vi "FGV_OBJ_login.vi"(6 "login_refnums":T1, 7 "options":T2, 8 "error_in":errorcluster, 9 "access_level_in":i32, 10 "username_in":string, 11 "ID_in":string) -> (0 "error_out":errorcluster, 1 "access_level_out":i32, 2 "username_out":string, 3 "ID_out":string, 5 "Login read active?":bool)   [LabVIEW 2020]
uses:
  FGV_OBJ_login.ctl
  OBJ_login_refnums.ctl
  test_button/FGV_OBJ_test_button.ctl
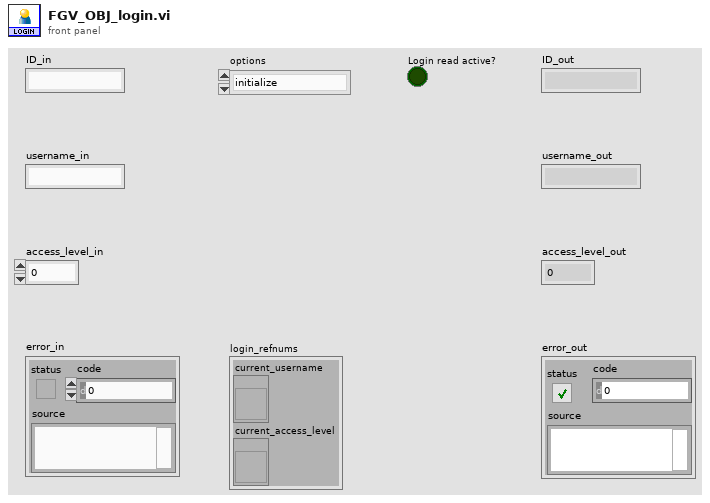
[diagram p1: front panel]
types:
  T1 = typedef "OBJ_login_refnums.ctl" = cluster{"current_username":refnum<vi>, "current_access_level":refnum<vi>}
  T2 = typedef "FGV_OBJ_login.ctl" = enum16{"initialize", "start_login_read", "end_login_read", "login", "logout", "get_login_info"}
  T3 = typedef "FGV_OBJ_test_button.ctl" = enum16{"initialize", "set_new_login", "set_message", "enable", "disable", "disable_gray", "translate", "set_scan_tooling", "get_scan_tooling"}
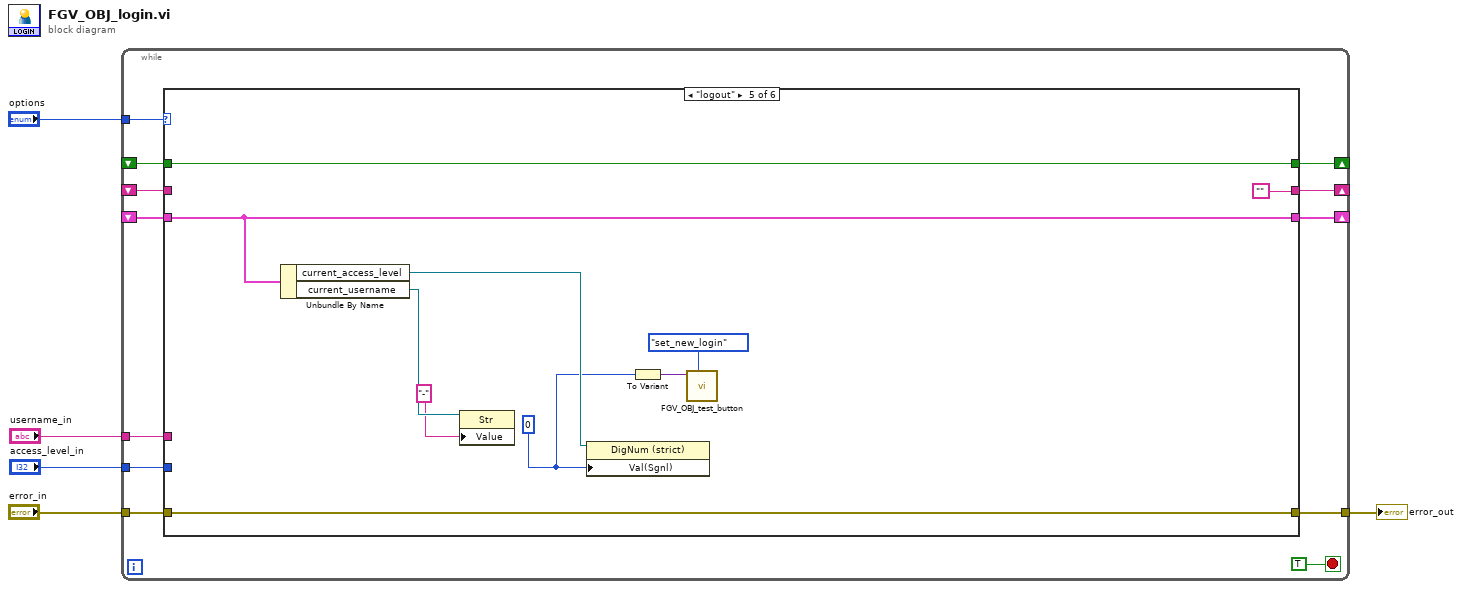
[diagram p0: block diagram]
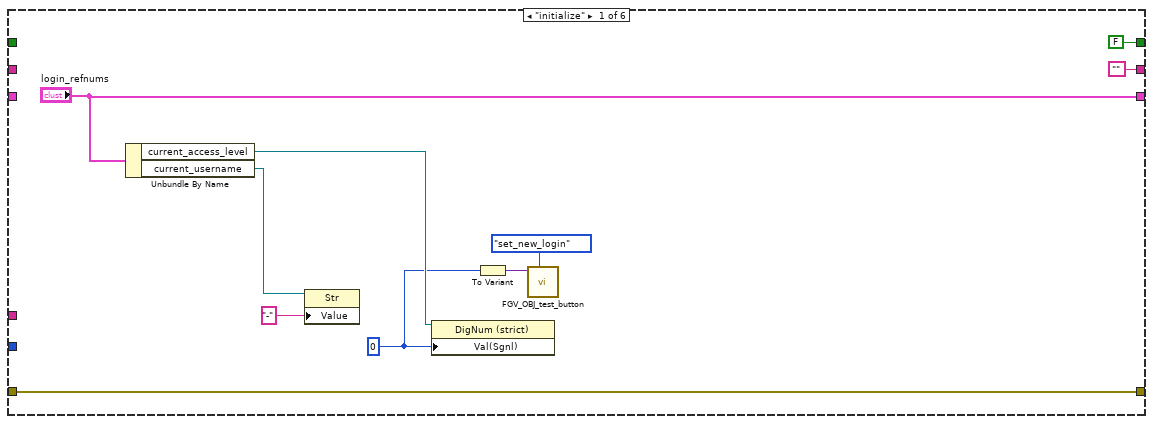
[diagram p2: hidden frame]
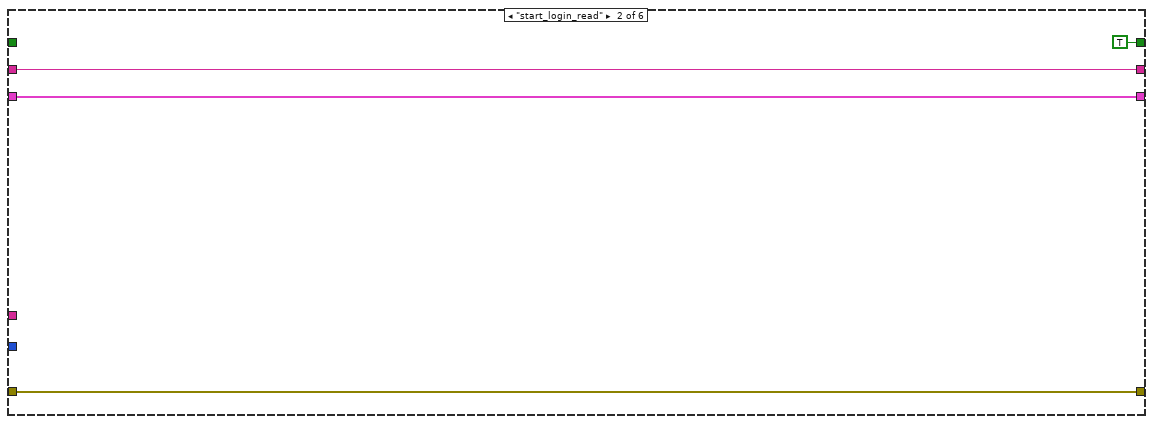
[diagram p3: hidden frame]
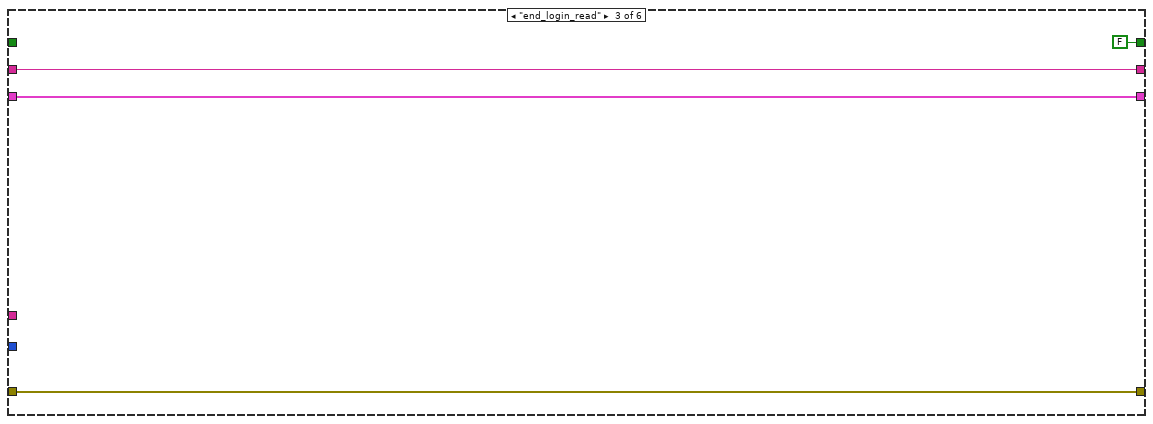
[diagram p4: hidden frame]
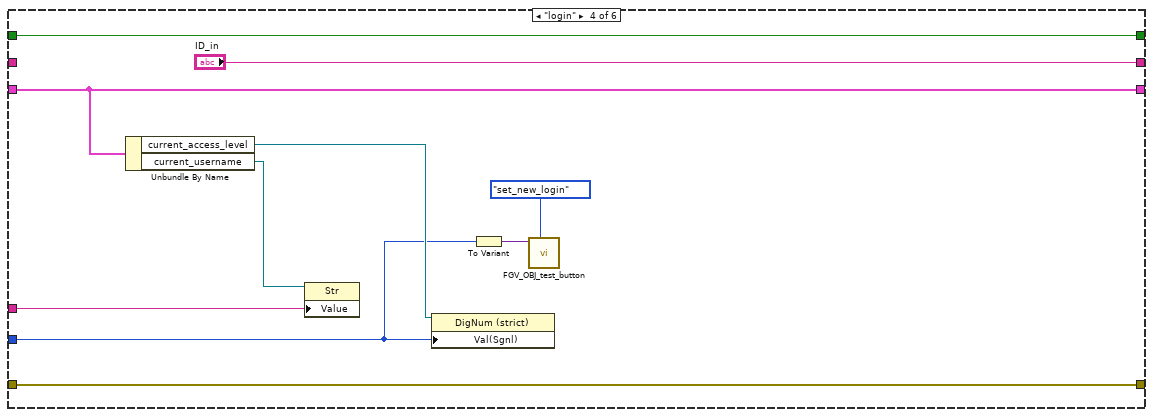
[diagram p5: hidden frame]
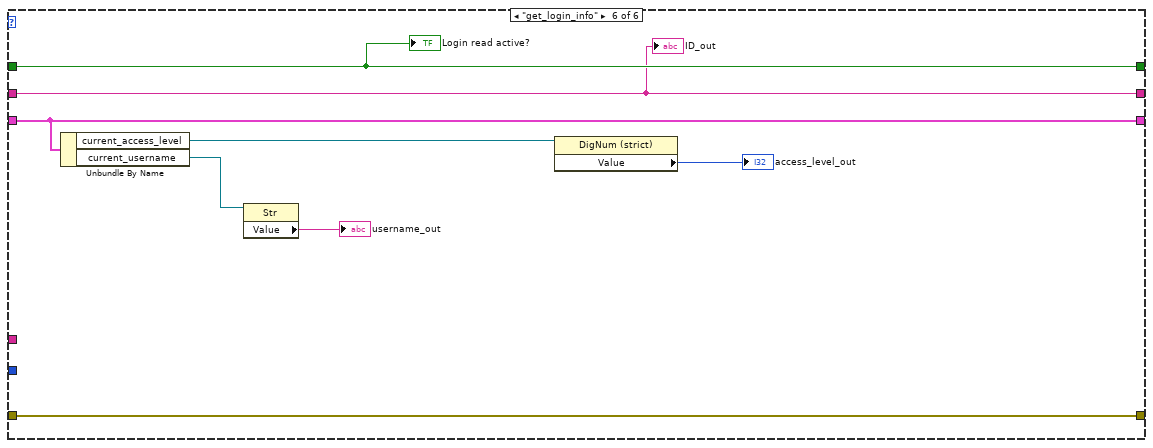
[diagram p6: hidden frame]
diagram:
  n1 = while {
    tunnel: "options" -> [w16]
    tunnel: [w15] -> w5
    tunnel: "error_in" -> [w14]
    shift-right: [w13] -> _
    shift-left: _ -> [w12]
    tunnel: "username_in" -> [w11]
    tunnel: "access_level_in" -> [w10]
    shift-right: [w9] -> _
    shift-left: _ -> [w8]
    shift-right: [w7] -> _
    shift-left: _ -> [w6]
    stop <- TRUE stop-if-true
    n2 = case shown="\"logout\"" w16 {
      tunnel: [w27 w31 w35 w45 w55 w63] -> w15
      tunnel: w14 -> [w27 w31 w35 w45 w55 w63]
      tunnel: ["login_refnums" w30 w32 w41 w51 w62] -> w13
      tunnel: w12 -> [_ w30 w32 w41 w51 w62]
      tunnel: w11 -> [_ _ _ w44 _ _]
      tunnel: w10 -> [_ _ _ w40 _ _]
      tunnel: ["" w29 w33 "ID_in" "" w56] -> w9
      tunnel: w8 -> [_ w29 w33 _ _ w56]
      tunnel: [FALSE TRUE FALSE w36 w46 w58] -> w7
      tunnel: w6 -> [_ _ _ w36 w46 w58]
      frame "initialize" {
        w22 = 0 ("Value")
        n3 = Unbundle By Name("login_refnums") -> ("current_access_level"=w25:refnum<vi>, "current_username"=w26:refnum<vi>)
        n4 = property class="Str"(reference=w26, "Value"="-") -> ()  [unwired: 1 in, 2 out]
        n5 = property class="DigNum (strict)"(reference=w25, "Val(Sgnl)"=w22) -> ()  [unwired: 1 in, 2 out]
        n6 = To Variant(anything=w22) -> (Variant=w19:variant)
        n7 = call "FGV_OBJ_test_button.vi"("options"=FGV_OBJ_test_button."set_new_login", "input"=w19) -> ()  [unwired: 8 in, 2 out]
      }
      frame "start_login_read" {
      }
      frame "end_login_read" {
      }
      frame "login" {
        n8 = Unbundle By Name(w41) -> ("current_access_level"=w42:refnum<vi>, "current_username"=w43:refnum<vi>)
        n9 = property class="Str"(reference=w43, "Value"=w44) -> ()  [unwired: 1 in, 2 out]
        n10 = property class="DigNum (strict)"(reference=w42, "Val(Sgnl)"=w40) -> ()  [unwired: 1 in, 2 out]
        n11 = To Variant(anything=w40) -> (Variant=w37:variant)
        n12 = call "FGV_OBJ_test_button.vi"("options"=FGV_OBJ_test_button."set_new_login", "input"=w37) -> ()  [unwired: 8 in, 2 out]
      }
      frame "logout" {
        w50 = 0 ("Value")
        n13 = Unbundle By Name(w51) -> ("current_access_level"=w53:refnum<vi>, "current_username"=w54:refnum<vi>)
        n14 = property class="Str"(reference=w54, "Value"="-") -> ()  [unwired: 1 in, 2 out]
        n15 = property class="DigNum (strict)"(reference=w53, "Val(Sgnl)"=w50) -> ()  [unwired: 1 in, 2 out]
        n16 = To Variant(anything=w50) -> (Variant=w47:variant)
        n17 = call "FGV_OBJ_test_button.vi"("options"=FGV_OBJ_test_button."set_new_login", "input"=w47) -> ()  [unwired: 8 in, 2 out]
      }
      frame "get_login_info" {
        n18 = Unbundle By Name(w62) -> ("current_access_level"=w60:refnum<vi>, "current_username"=w61:refnum<vi>)
        n19 = property class="Str"(reference=w61) -> ("Value"=→"username_out":string)  [unwired: 1 in, 2 out]
        n20 = property class="DigNum (strict)"(reference=w60) -> ("Value"=→"access_level_out":i32)  [unwired: 1 in, 2 out]
        "Login read active?" <- w58
        "ID_out" <- w56
      }
    }
  }
  "error_out" <- w5
